vi "Get Read Position.vi"(8 "error in (no error)":errorcluster, 11 "StringStream in":refnum<class "StringStream.lvclass">) -> (0 "error out":errorcluster, 2 "Read Position":i64, 3 "StringStream out":refnum<class "StringStream.lvclass">)   [LabVIEW 2020, in "IO.lvlib" / "StringStream.lvclass"]
uses:
  StringStream.lvclass
  StringStream.lvclass/StringStream.ctl
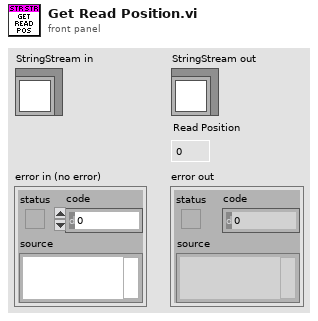
[diagram p1: front panel]
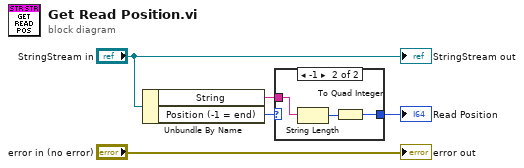
[diagram p0: block diagram]
diagram:
  n1 = Unbundle By Name("StringStream in") -> ("String"=w4:string, "Position (-1 = end)"=w5:i64)
  n2 = case shown="-1" w5 {
    selector: w5 -> [w6 _]
    tunnel: w4 -> [_ w9]
    tunnel: [w6 w7] -> w3
    frame Default {
    }
    frame -1 {
      n3 = String Length(string=w9) -> (length=w8:i32)
      n4 = To Quad Integer(1:w8) -> (0:w7:i64)
    }
  }
  "Read Position" <- w3
  "error out" <- "error in (no error)"
  "StringStream out" <- "StringStream in"
